vi "System Parameters.vi"(8 "Error In":errorcluster, 11 "System Spec Widget in":refnum<class "System Spec Widget.lvclass">) -> (0 "Error Out":errorcluster, 2 "System Parameters":T1, 3 "System Spec Widget out":refnum<class "System Spec Widget.lvclass">)   [LabVIEW 2014, in "System Spec Widget.lvclass"]
doc: "Gets the parameters that the user has inputted.\n\n\nCopyright (c) 2019 Sze Howe Koh.\nThis code is licensed under the MIT license."
uses:
  System Spec Widget.lvclass
  System Parameters.ctl
  System Spec Widget.lvclass/System Spec Widget.ctl
  <vilib>/addons/LQ/Qt Widgets/QSpinBox/QSpinBox.lvclass
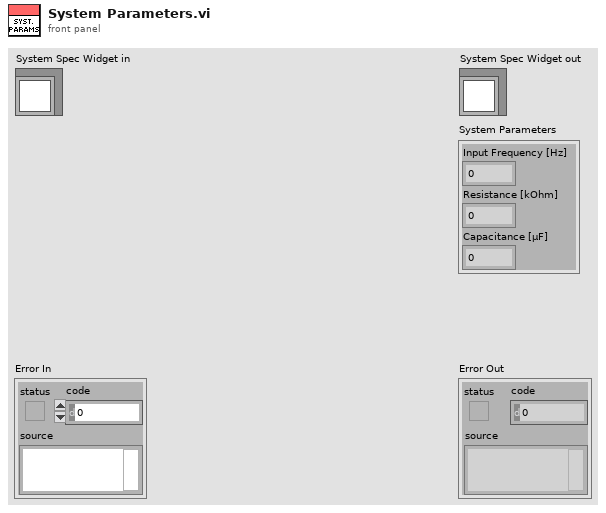
[diagram p1: front panel]
types:
  T1 = typedef "System Spec Widget.lvclass/System Parameters.ctl" = cluster{"Input Frequency [Hz]":i32, "Resistance [kOhm]":i32, "Capacitance [µF]":i32}
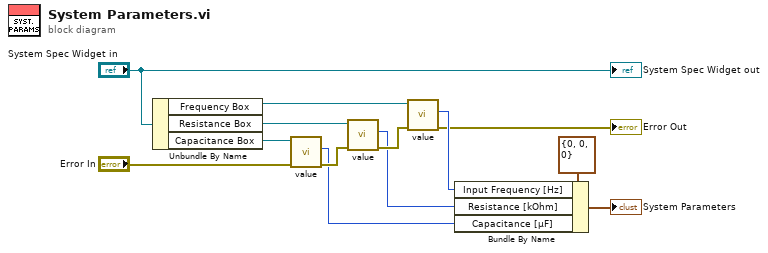
[diagram p0: block diagram]
diagram:
  n1 = Unbundle By Name("System Spec Widget in") -> ("Frequency Box"=w11:refnum<class "QSpinBox.lvclass">, "Resistance Box"=w10:refnum<class "QSpinBox.lvclass">, "Capacitance Box"=w9:refnum<class "QSpinBox.lvclass">)
  n2 = call <vilib>:"value.vi"("Error In"="Error In", "QSpinBox In"=w9) -> ("Error Out"=w8:errorcluster, "Value"=w6:i32)  [unwired: 7 in, 1 out]
  n3 = call <vilib>:"value.vi"("Error In"=w8, "QSpinBox In"=w10) -> ("Error Out"=w7:errorcluster, "Value"=w5:i32)  [unwired: 7 in, 1 out]
  n4 = call <vilib>:"value.vi"("Error In"=w7, "QSpinBox In"=w11) -> ("Error Out"=→"Error Out":errorcluster, "Value"=w4:i32)  [unwired: 7 in, 1 out]
  n5 = Bundle By Name(cluster=T1 {"Input Frequency [Hz]"=0, "Resistance [kOhm]"=0, "Capacitance [µF]"=0} ("System Parameters"), "Input Frequency [Hz]"=w4, "Resistance [kOhm]"=w5, "Capacitance [µF]"=w6) -> (→"System Parameters":T1)
  "System Spec Widget out" <- "System Spec Widget in"
